vi "Write_Datafile.vi"(8 "error in (no error)":errorcluster, 10 "Dynamic data":T1, 11 "Input parameters":T2={"Measurement type"=enum."Debug", "Sensor type"=enum."HPK_8in_256", "Identifier"="test.txt", "Open after execution?"=FALSE, "Plot after execution?"=FALSE, "Display channel"=0, "Voltage Delay (s)"=0.5, "Switch Delay (s)"=0.01, "VISA resource name source"="", "VISA resource name DMM"="", "VISA resource name LCR"="", "Compliance  Level (uA)"=10.0, "Voltage Limit (V)"=1000.0, "Data storage location"="", "Scan voltages"="", "Use source as DMM?"=FALSE, "LCR signal frequenzy (Hz)"=10.0, "DMM device"=enum."Keithley2001", "Sampling number"=1, "Use env. sensors on"=enum."Sensirion sht1x/7x", "Switchboard Handle"=0, "Use Switchboard"=FALSE, "LCR signal voltage (V)"=10000.0, "Repeat"=1, "Test Run Limit (nA)"=10.0, "Scan voltages IV"="", "Scan voltages CV"="", "Hex pad numbers?"=FALSE, "Set measurement type"=enum."Debug", "Custom pad scan"="", "IV voltage Delay (s)"=0.5, "CV voltage Delay (s)"=0.5} {"CV voltage Delay (s)" format="%#_13g"; "IV voltage Delay (s)" format="%#_13g"; "Voltage Limit (V)" format="%#_13g"; "Voltage Delay (s)" format="%#_13g"; "Switch Delay (s)" format="%#_13g"}) -> (0 "error out":errorcluster, 2 "Text":string, 3 "File path":path)   [LabVIEW 2016]
uses:
  Input_parameters.ctl
  Dynamic_data.ctl
  <vilib>/Utility/file.llb/Write Delimited Spreadsheet (string).vi
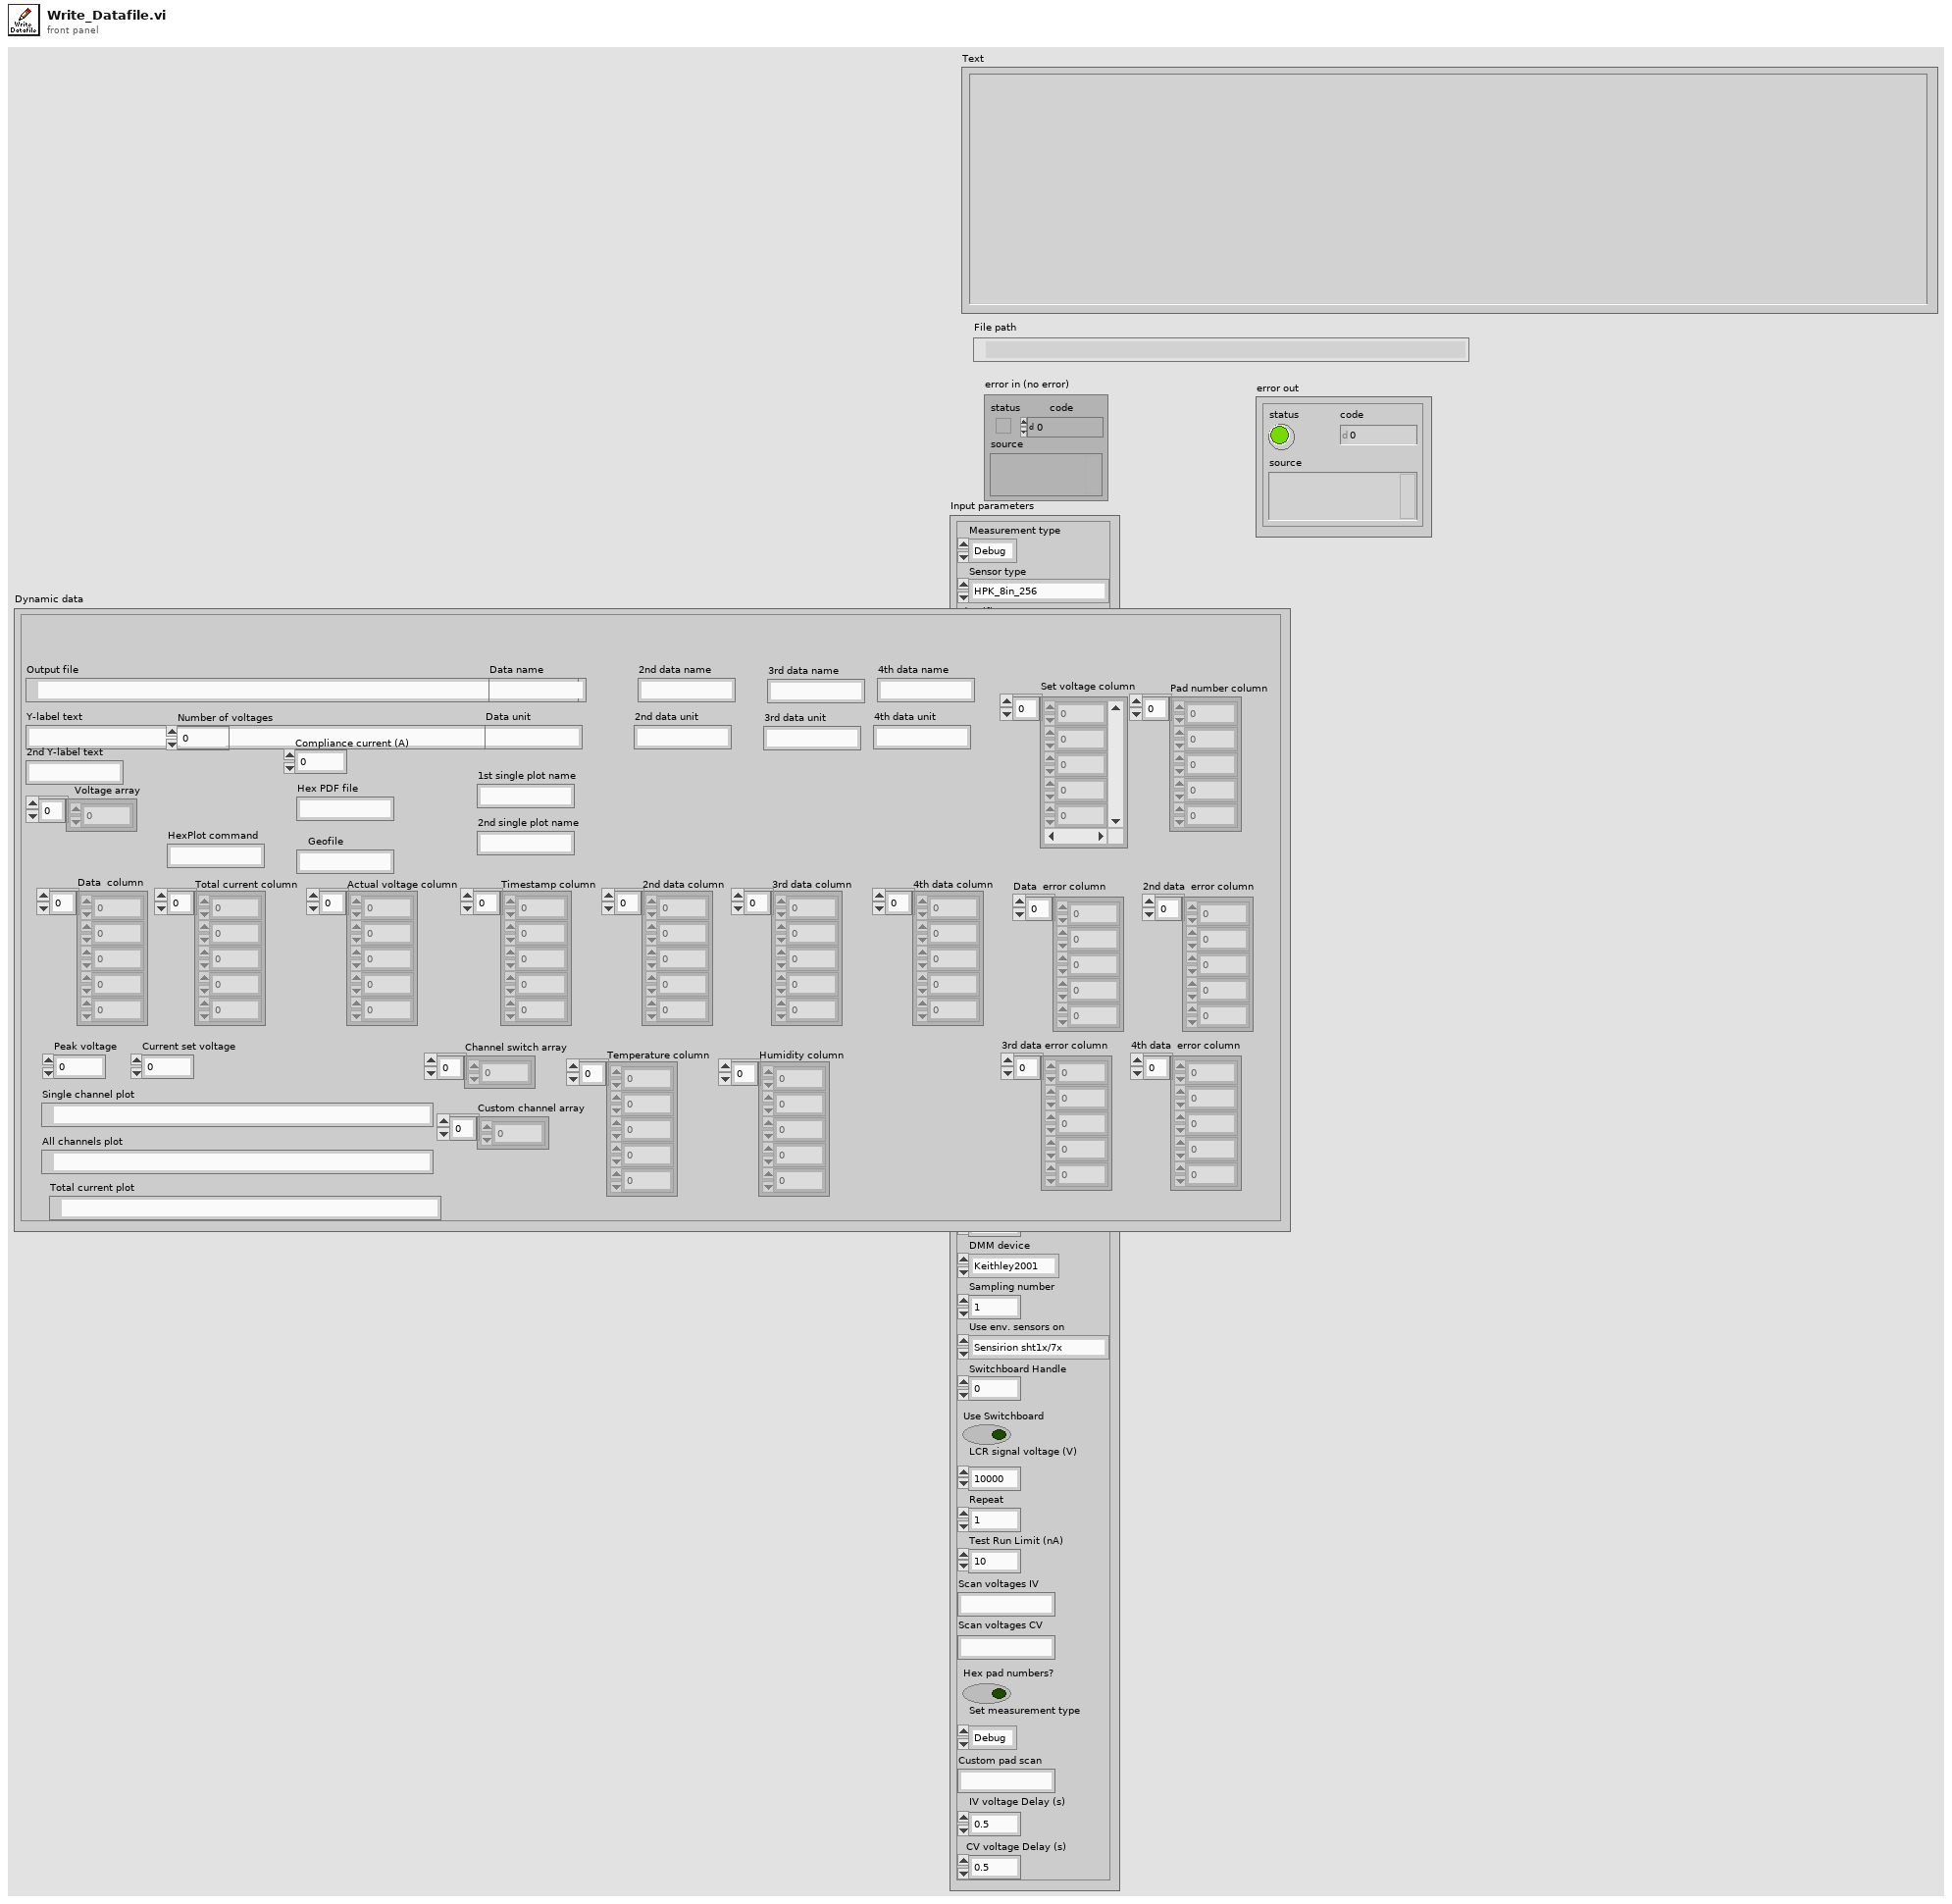
[diagram p1: front panel]
types:
  T1 = typedef "Dynamic_data.ctl" = cluster{"Output file":path, "Y-label text":string, "Current set voltage":dbl, "Set voltage column":dbl[], "Pad number column":dbl[], "Data  column":dbl[], "Number of voltages":i32, "Compliance current (A)":dbl, "Geofile":string, "Peak voltage":dbl, "Hex PDF file":string, "Voltage array":dbl[], "Total current column":dbl[], "Timestamp column":dbl[], "Data name":string, "Data unit":string, "2nd data column":dbl[], "2nd data name":string, "2nd data unit":string, "3rd data column":dbl[], "4th data column":dbl[], "3rd data name":string, "3rd data unit":string, "4th data name":string, "4th data unit":string, "Actual voltage column":dbl[], "2nd Y-label text":string, "Single channel plot":path, "Temperature column":dbl[], "Humidity column":dbl[], "Channel switch array":i32[], "1st single plot name":string, "2nd single plot name":string, "All channels plot":path, "HexPlot command":string, "Custom channel array":i32[], "Data  error column":dbl[], "2nd data  error column":dbl[], "3rd data error column":dbl[], "4th data  error column":dbl[], "Total current plot":path}
  T2 = typedef "Input_parameters.ctl" = cluster{"Measurement type":enum16{"IV", "CV", "Debug", "Test"}, "Sensor type":enum16{"HPK_6in_135", "HPK_8in_256", "INF_8in_256", "Diode", "HPK_6in_256", "Test capacitances", "Full matrix"}, "Identifier":string, "Open after execution?":bool, "Plot after execution?":bool, "Display channel":i32, "Voltage Delay (s)":dbl, "Switch Delay (s)":dbl, "VISA resource name source":refnum<visa-resource-name>, "VISA resource name DMM":refnum<visa-resource-name>, "VISA resource name LCR":refnum<visa-resource-name>, "Compliance  Level (uA)":dbl, "Voltage Limit (V)":dbl, "Data storage location":string, "Scan voltages":string, "Use source as DMM?":bool, "LCR signal frequenzy (Hz)":dbl, "DMM device":enum16{"Keithley2001", "Keithley2450", "Keithley2410", "Keithley6487"}, "Sampling number":i32, "Use env. sensors on":enum16{"Sensirion sht1x/7x", "Switch Matrix", "Probecard"}, "Switchboard Handle":u32, "Use Switchboard":bool, "LCR signal voltage (V)":dbl, "Repeat":i32, "Test Run Limit (nA)":dbl, "Scan voltages IV":string, "Scan voltages CV":string, "Hex pad numbers?":bool, "Set measurement type":enum16{"IV", "CV", "Debug", "Test", "IV+CV"}, "Custom pad scan":string, "IV voltage Delay (s)":dbl, "CV voltage Delay (s)":dbl}
  T3 = enum16{"HPK_6in_135", "HPK_8in_256", "INF_8in_256", "Diode", "HPK_6in_256", "Test capacitances", "Full matrix"}
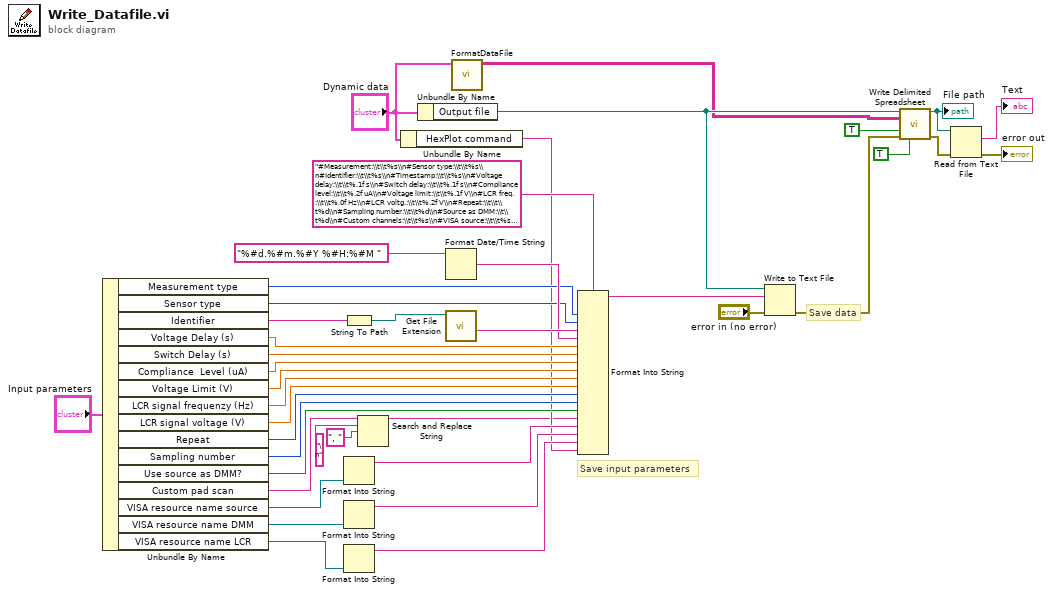
[diagram p0: block diagram]
diagram:
  # "Save data"
  # "Save input parameters"
  n1 = Unbundle By Name("Input parameters") -> ("Measurement type"=w34:enum16{"IV", "CV", "Debug", "Test"}, "Sensor type"=w33:T3, "Identifier"=w32:string, "Voltage Delay (s)"=w31:dbl, "Switch Delay (s)"=w30:dbl, "Compliance  Level (uA)"=w29:dbl, "Voltage Limit (V)"=w28:dbl, "LCR signal frequenzy (Hz)"=w26:dbl, "LCR signal voltage (V)"=w25:dbl, "Repeat"=w23:i32, "Sampling number"=w24:i32, "Use source as DMM?"=w27:bool, "Custom pad scan"=w2:string, "VISA resource name source"=w22:refnum<visa-resource-name>, "VISA resource name DMM"=w21:refnum<visa-resource-name>, "VISA resource name LCR"=w20:refnum<visa-resource-name>)
  n2 = String To Path(string=w32) -> (path=w39:path)
  n3 = Format Into String(w22) -> (resulting string=w19:string)  [unwired: 3 in, 1 out]
  n4 = Format Into String(w21) -> (resulting string=w18:string)  [unwired: 3 in, 1 out]
  n5 = Format Into String(w20) -> (resulting string=w17:string)  [unwired: 3 in, 1 out]
  n6 = Search and Replace String(input string=w2, search string="\n", replace string=", " ("replace string (\"\")")) -> (result string=w1:string)  [unwired: 5 in, 3 out]
  n7 = Unbundle By Name("Dynamic data") -> ("HexPlot command"=w5:string)
  n8 = Unbundle By Name("Dynamic data") -> ("Output file"=w13:path)
  n9 = Format Date/Time String(time format string (%c)="%#d.%#m.%#Y %#H:%#M ") -> (date/time string=w36:string)  [unwired: 2 in]
  n10 = call <vilib>:"Get File Extension.vi"("file"=w39) -> ("filename without extension"=w38:string)  [unwired: 6 in, 4 out]
  n11 = call "FormatDataFile.vi"("Dynamic data"="Dynamic data") -> ("appended array"=w12:string[][])  [unwired: 10 in]
  n12 = Format Into String(format string="#Measurement:\\t\\t%s\\n#Sensor type:\\t\\t%s\\n#Identifier:\\t\\t%s\\n#Timestamp:\\t\\t%s\\n#Voltage delay:\\t\\t%.1f s\\n#Switch delay:\\t\\t%.1f s\\n#Compliance level:\\t\\t%.2f uA\\n#Voltage limit:\\t\\t%.1f V\\n#LCR freq.:\\t\\t%.0f Hz\\n#LCR voltg.:\\t\\t%.2f V\\n#Repeat:\\t\\t\\t%d\\n#Sampling number:\\t\\t%d\\n#Source as DMM:\\t\\t%d\\n#Custom channels:\\t\\t%s\\n#VISA source:\\t\\t%s\\n#VISA DMM:\\t\\t%s\\n#VISA LCR:\\t\\t%s\\n#HexPlot cmd:\\t\\t%s\\n\\n", w34, w33, w38, w36, w31, w30, w29, w28, w26, w25, w23, w24, w27, w1, w19, w18, w17, w5) -> (resulting string=w40:string)  [unwired: 2 in, 1 out]
  n13 = Write to Text File(file (use dialog)=w13, text=w40, error in="error in (no error)") -> (error out=w11:errorcluster)  [unwired: 1 in, 2 out]
  n14 = call-poly <vilib>:"Write Delimited Spreadsheet.vi"("file path (dialog if empty)"=w13, "2D data"=w12, "append to file? (new file:F)"=TRUE, "error in (no error)"=w11, "transpose? (no:F)"=TRUE) -> ("new file path (Not A Path if cancelled)"=w8:path, "error out"=w10:errorcluster)  [unwired: 9 in]
  "File path" <- w8
  n15 = Read from Text File(file (use dialog)=w8, error in=w10) -> (text=→"Text":string, error out=→"error out":errorcluster)  [unwired: 2 in, 2 out]
